vi "Plot.vi"(11 "AER in":refnum<class "AER.lvclass">) -> ()   [LabVIEW 2016, in "AER.lvclass"]
uses:
  AER.lvclass
  <vilib>/Utility/miscctls.llb/LVBoundsTypeDef.ctl
  Controls/Neuron Info.ctl
  Controls/Type of Neuron.ctl
  AER.lvclass/AER.ctl
panel:
  out "No Neurons":i32
  in  "Stop Button":bool
  out "NoPre [i]":i32
  in  "N":i32
  out "2D Picture":picture
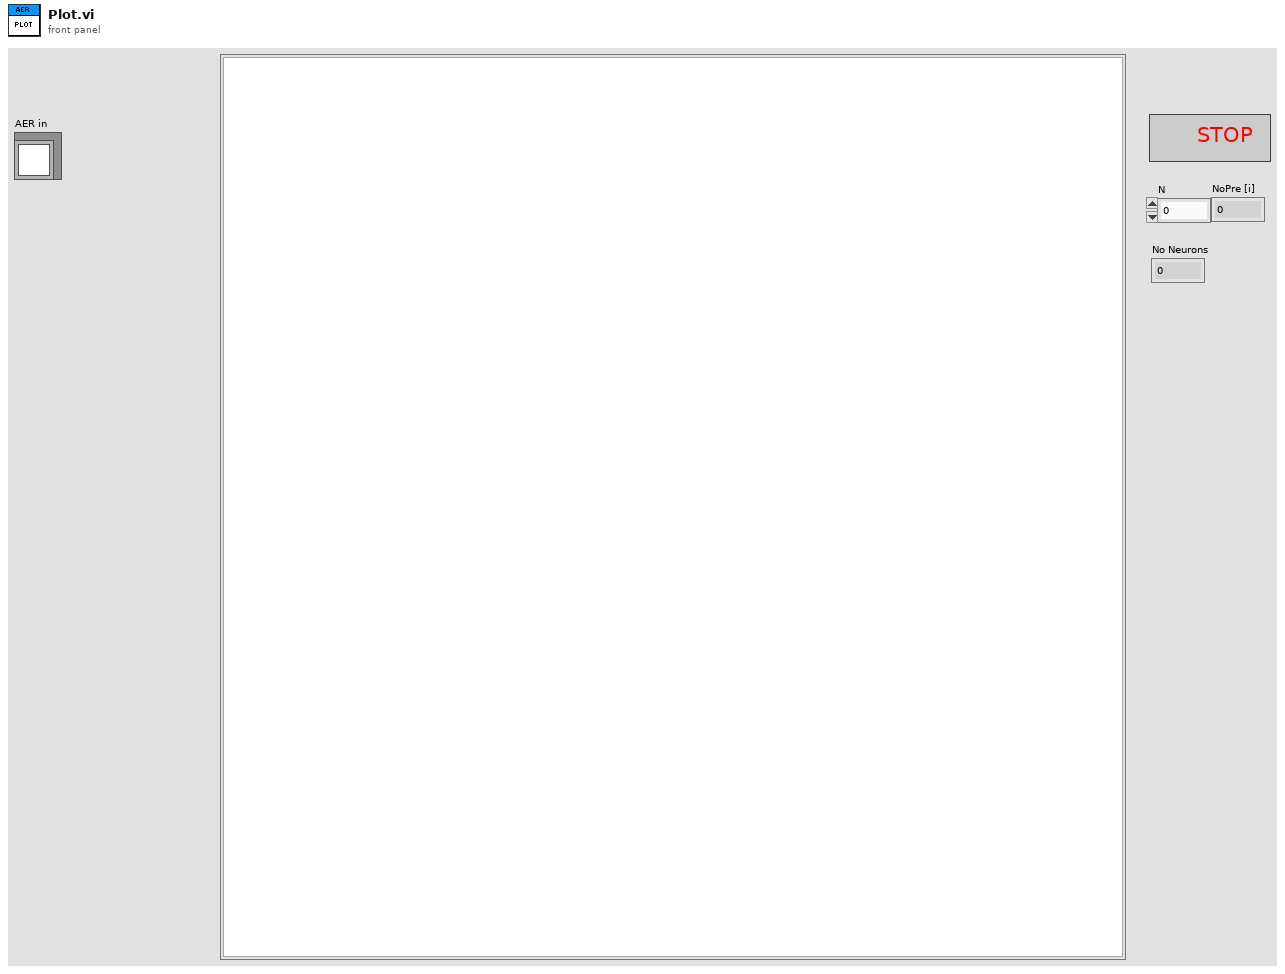
[diagram p1: front panel]
types:
  T1 = typedef "Neuron Info.ctl" = cluster{"N":i32, "Radius":dbl, "Type":T2, "Color":u32}[]
  T2 = typedef "Type of Neuron.ctl" = enum16{"MF", "BA", "GO", "GC", "PC", "LU", "Glia (Dummy)"}
  T3 = typedef "LVBoundsTypeDef.ctl" = cluster{"Width":u32, "Height":u32}
  T4 = cluster{"Width":u16, "Style":enum32{"Solid", "Dash", "Dot", "DashDot", "DashDotDot"}}
  T5 = enum32{"Solid", "Dash", "Dot", "DashDot", "DashDotDot"}
  T6 = cluster{dbl, "Style":enum32{"Solid", "Dash", "Dot", "DashDot", "DashDotDot"}}
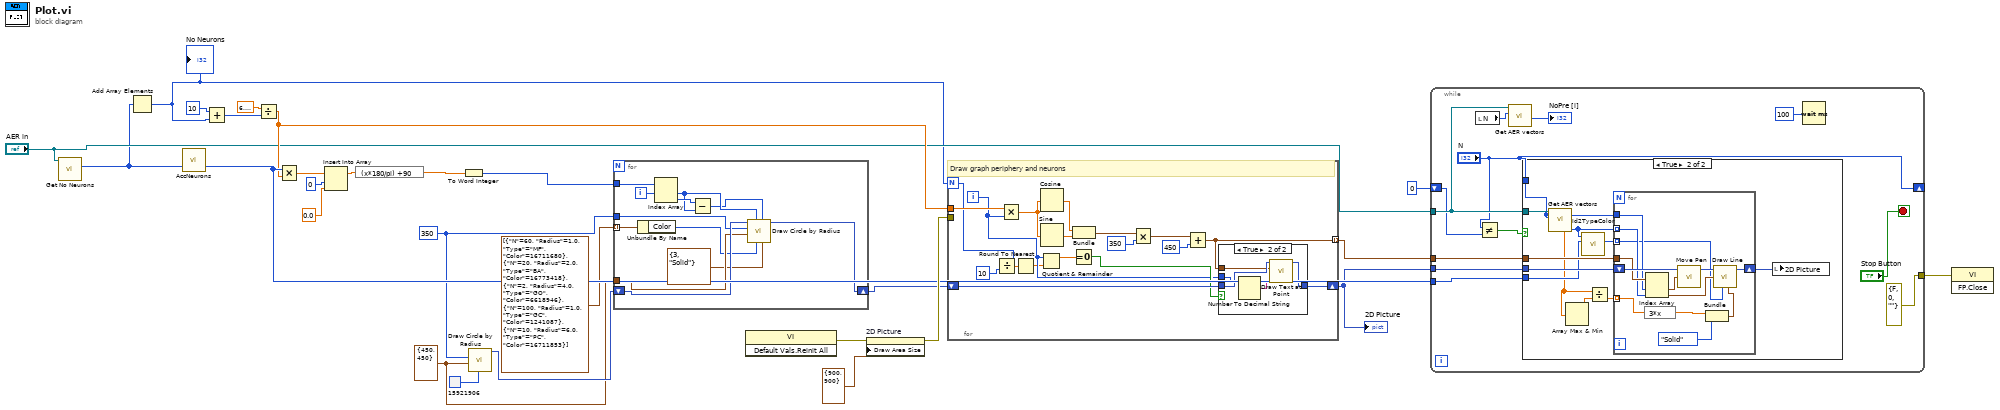
[diagram p0: block diagram]
diagram:
  w16 = cluster{"horizontal":i16, "vertical":i16} {"horizontal"=450, "vertical"=450} ("pixel center")
  w15 = i16 350 ("radius")
  n1 = call "Get No Neurons.vi"("AER in"="AER in") -> ("No N"=w4:i32[])  [unwired: 9 in, 1 out]
  n2 = Add Array Elements(numeric array=w4) -> (sum=w3:i32)
  "No Neurons" <- w3
  n3 = call "AccNeurons.vi"("No N"=w4) -> ("No N acc"=w19:i32[])  [unwired: 2 in]
  n4 = Add(x=10, y=w3) -> (x+y=w20:i32)
  n5 = Divide(x=6.283185307179586, y=w20) -> (x/y=w6:dbl)
  n6 = Multiply(x=w19, y=w6) -> (x*y=w11:dbl[])
  n7 = Insert Into Array(array=w11, index=0, new element=0.0 ("new element/subarray")) -> (w10:dbl[])
  n8 = expression code="(x*180/pi) +90"(w10) -> (w9:dbl[])
  n9 = To Word Integer(number=w9) -> (16bit integer=w7:i16[])
  n10 = call <vilib>:"Draw Circle by Radius.vi"("color(black)"=u32 15921906, "pixel center"=w16, "radius"=w15) -> ("new picture"=w17:picture)  [unwired: 8 in]
  n11 = for {
    tunnel: w16 -> [w38]
    tunnel: w15 -> [w37]
    tunnel: w7 -> [w34]
    tunnel: T1 [{"N"=60, "Radius"=1.0, "Type"=enum."MF", "Color"=16711680}, {"N"=20, "Radius"=2.0, "Type"=enum."BA", "Color"=16773418}, {"N"=2, "Radius"=4.0, "Type"=enum."GO", "Color"=6618946}, {"N"=100, "Radius"=1.0, "Type"=enum."GC", "Color"=1241087}, {"N"=10, "Radius"=6.0, "Type"=enum."PC", "Color"=16711853}] ("Neurons Info") -> [w32] mode=indexing
    shift-right: [w36] -> w14
    shift-left: w17 -> [w39]
    i -> [w33]
    n12 = Unbundle By Name(w32) -> ("Color"=w31:u32)
    n13 = Index Array(array=w34, index #1=w33) -> (element #1=w29:i16, element #2=w30:i16)  [unwired: 1 in]
    n14 = Subtract(x=w30, y=w29) -> (x-y=w28:i16)
    n15 = call <vilib>:"Draw Circle by Radius.vi"("pen"=T4 {"Width"=3, "Style"=enum."Solid"}, "arc size(360)"=w28, "color(black)"=w31, "start angle(0)"=w29, "pixel center"=w38, "radius"=w37, "picture"=w39) -> ("new picture"=w36:picture)  [unwired: 4 in]
  }
  n16 = invoke class="VI" method="Default Vals.Reinit All"() -> (error out=w23:errorcluster)  [unwired: 3 in, 2 out]
  n17 = property on="2D Picture" class="Pict"(error in=w23, "Draw Area Size"=T3 {"Width"=900, "Height"=900}) -> (error out=w25:errorcluster)  [unwired: 1 in, 1 out]
  n18 = for {
    N: w3 -> [w44]
    shift-right: [w49] -> w18
    shift-left: w14 -> [w53]
    tunnel: w6 -> [w52]
    tunnel: [w50] -> w24 mode=indexing
    tunnel: w25 -> [_]
    i -> [w41]
    # "Draw graph periphery and neurons"
    n19 = Divide(x=w44, y=10 ("x")) -> (x/y=w43:dbl)
    n20 = Multiply(x=w52, y=w41) -> (x*y=w47:dbl)
    n21 = Round To Nearest(number=w43) -> (nearest integer value=w40:dbl)
    n22 = Quotient & Remainder(x=w41, y=w40) -> (x-y*floor(x/y)=w46:dbl)  [unwired: 1 out]
    n23 = Cosine(x=w47) -> (cos(x)=w48:dbl)
    n24 = Sine(x=w47) -> (sin(x)=w57:dbl)
    n25 = Equal To 0?(x=w46) -> (x = 0?=w45:bool)
    n26 = Bundle(w48, w57) -> (w51:cluster{dbl, dbl})  [unwired: 1 in]
    n27 = Multiply(x=w51, y=i16 350 ("vertical")) -> (x*y=w56:cluster{dbl, dbl})
    n28 = Add(x=w56, y=i16 450 ("vertical")) -> (x+y=w50:cluster{dbl, dbl})
    n29 = case shown="True" w45 {
      tunnel: w53 -> [w58 w63]
      tunnel: [w58 w62] -> w49
      tunnel: w41 -> [_ w61]
      tunnel: w50 -> [_ w59]
      frame False {
      }
      frame True {
        n30 = Number To Decimal String(number=w61) -> (decimal integer string=w60:string)  [unwired: 1 in]
        n31 = call <vilib>:"Draw Text at Point.vi"("text"=w60, "origin"=w59, "picture"=w63) -> ("new picture"=w62:picture)  [unwired: 7 in, 1 out]
      }
    }
  }
  "2D Picture" <- w18
  n32 = while {
    tunnel: "AER in" -> [w73]
    tunnel: w24 -> [w75]
    tunnel: w18 -> [w74]
    tunnel: w19 -> [w70]
    shift-right: ["N"] -> _
    shift-left: 0 ("N") -> [w68]
    tunnel: [errorcluster {"status"=FALSE, "code"=0, "source"=""} ("error constant")] -> w1
    stop <- "Stop Button" stop-if-true
    n33 = local read "N"() -> (w71:i32)
    n34 = Not Equal?(x="N", y=w68) -> (x != y?=w69:bool)
    n35 = call "Get AER vectors.vi"("ID [i]"=w71, "AER in"=w73) -> ("NoPre [i]"=→"NoPre [i]":i32)  [unwired: 4 in, 5 out]
    n36 = case shown="True" w69 {
      tunnel: w75 -> [_ w86]
      tunnel: w74 -> [_ w85]
      tunnel: w73 -> [_ w84]
      tunnel: w70 -> [_ w83]
      tunnel: "N" -> [_ w82]
      frame False {
      }
      frame True {
        n37 = call "Get AER vectors.vi"("ID [i]"=w82, "AER in"=w84) -> ("PreIDs [i]"=w80:i32[], "W[i]"=w78:dbl[])  [unwired: 4 in, 4 out]
        n38 = Array Max & Min(array=w78) -> (max value=w76:dbl)  [unwired: 3 out]
        n39 = call "Id2TypeColor.vi"("Acc N"=w83, "PreIds"=w80) -> ("Colors"=w79:u32[])  [unwired: 8 in, 1 out]
        n40 = Divide(x=w78, y=w76) -> (x/y=w77:dbl[])
        n41 = for {
          tunnel: w80 -> [w92] mode=indexing
          tunnel: w86 -> [w96]
          shift-right: [w97] -> w81
          shift-left: w85 -> [w99]
          tunnel: w82 -> [w95]
          tunnel: w79 -> [w91] mode=indexing
          tunnel: w77 -> [w89] mode=indexing
          n42 = expression code="3*x"(w89) -> (w88:dbl)
          n43 = Index Array(array=w96, index #1=w95, index #2=w92) -> (element #1=w94:cluster{dbl, dbl}, element #2=w93:cluster{dbl, dbl})
          n44 = call <vilib>:"Move Pen.vi"("new position"=w94, "picture"=w99) -> ("new picture"=w98:picture)  [unwired: 3 in]
          n45 = Bundle(w88, "Style"=T5."Solid") -> (w90:T6)  [unwired: 1 in]
          n46 = call <vilib>:"Draw Line.vi"("picture"=w98, "end point"=w93, "color(black)"=w91, "pen"=w90) -> ("new picture"=w97:picture)  [unwired: 5 in]
        }
        n47 = local write "2D Picture"(w81) -> ()
      }
    }
    n48 = Wait (ms)(milliseconds to wait=u32 100) -> ()  [unwired: 1 out]
  }
  n49 = invoke class="VI" method="FP.Close"(error in=w1) -> ()  [unwired: 2 in, 3 out]
